vi "RetrievemeasurementByID.vi"(8 "error in (no error)":errorcluster, 10 "DatabaseConnectionInfo":T1, 11 "ID":string) -> (0 "error out":errorcluster, 1 "Variant data":variant[][](array[variant]), 2 "Double data":dbl[][](array[numeric]), 3 "String data":string[][](array[string]))   [LabVIEW 2017]
uses:
  <vilib>/addons/database/Connection.llb/DB Tools Open Connec (Path).vi
  <vilib>/addons/database/Connection.llb/Conn Execute.vi
  <vilib>/addons/database/Recordset.llb/Rec Fetch Recordset Data (R).vi
  <vilib>/addons/database/Recordset.llb/Rec Destroy - Connection.vi
  <vilib>/addons/database/_DB Variant To Data/Database Variant To Data.xnode
  <vilib>/addons/database/NI_Database_API.lvlib
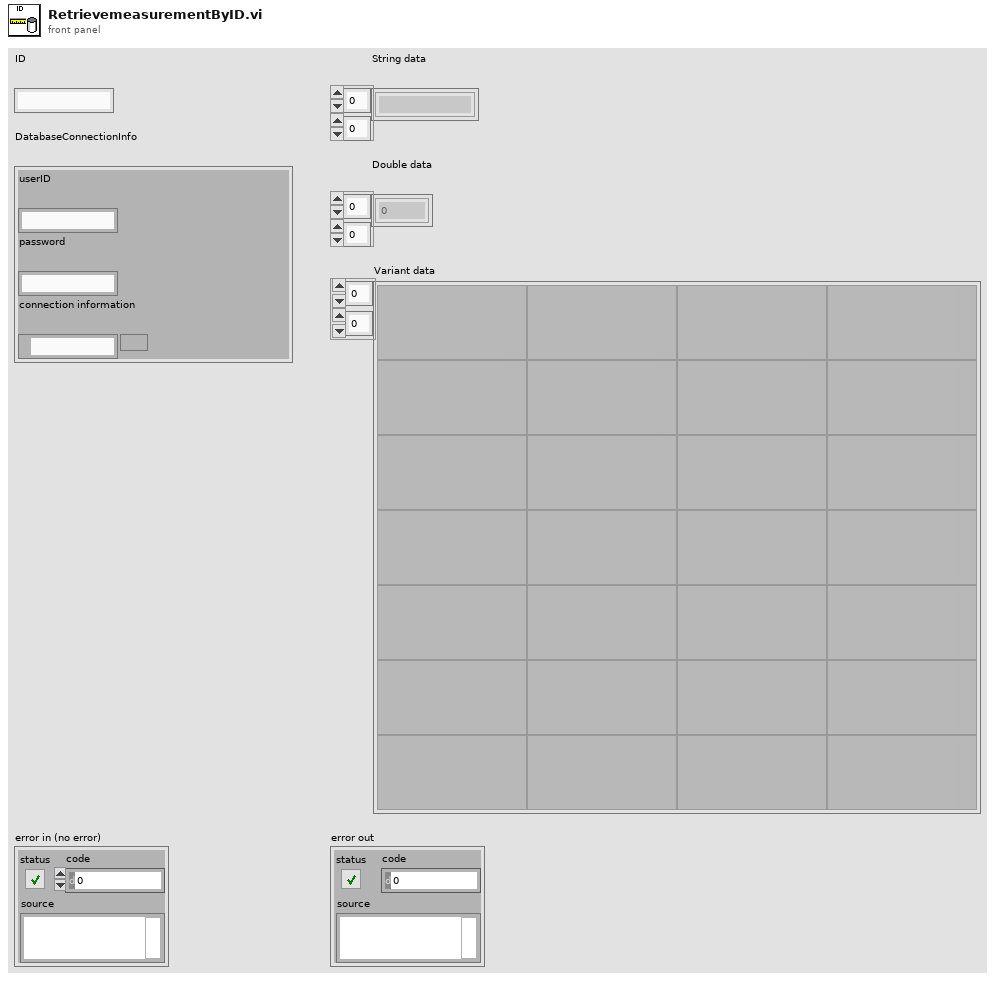
[diagram p1: front panel]
types:
  T1 = cluster{"userID":string, "password":string, "connection information":path}
  T2 = typedef "NI_Database_API.lvlib/Conn ObjectReference.ctl" = refnum<k1>
  T3 = typedef "NI_Database_API.lvlib/Rec ObjectReference.ctl" = refnum<k1>
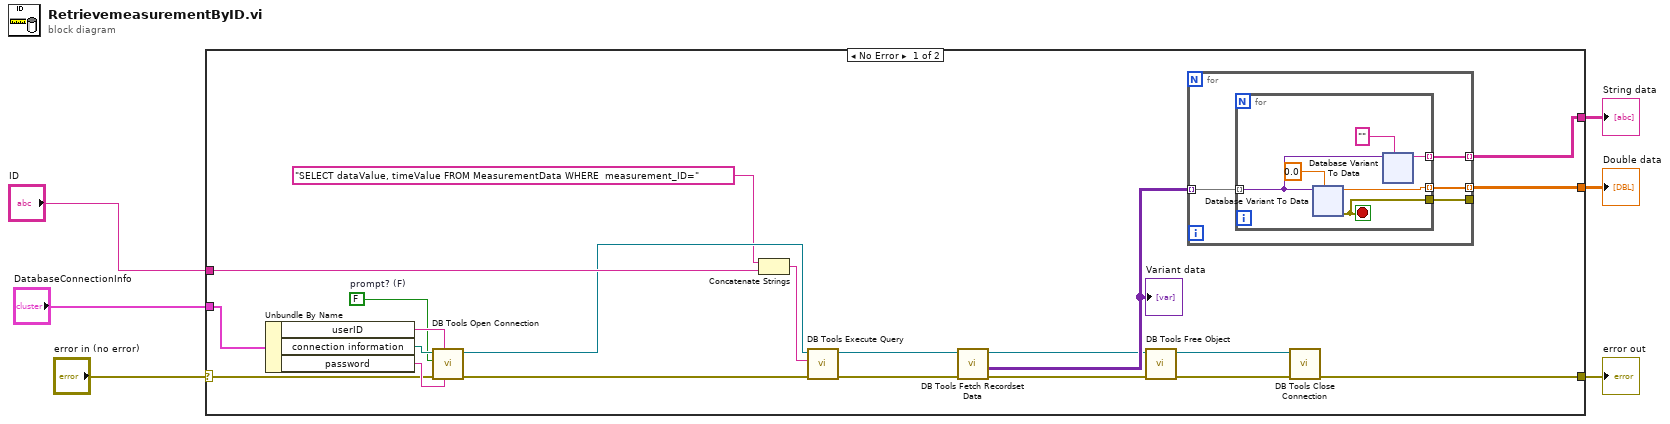
[diagram p0: block diagram]
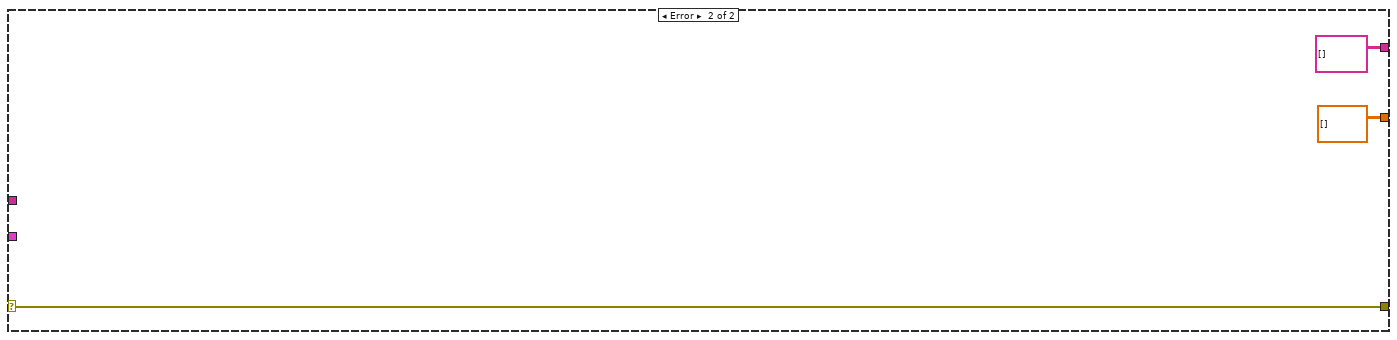
[diagram p2: hidden frame]
diagram:
  n1 = case shown="No Error" "error in (no error)" {
    selector: "error in (no error)" -> [w7 w104]
    tunnel: [w27 dbl[][] []] -> w6
    tunnel: [w26 string[][] []] -> w5
    tunnel: "ID" -> [w23 _]
    tunnel: "DatabaseConnectionInfo" -> [w22 _]
    tunnel: [w17 w104] -> w2
    frame No Error {
      w9 = FALSE  # prompt? (F)
      n2 = Unbundle By Name(w22) -> ("userID"=w10:string, "connection information"=w12:path, "password"=w11:string)
      n3 = call-poly <vilib>:"DB Tools Open Connection.vi"("password"=w11, "userID"=w10, "error in (no error)"=w7, "prompt? (F)"=w9, "connection information"=w12) -> ("error out"=w14:errorcluster, "connection reference"=w13:T2)  [unwired: 3 in]
      n4 = Concatenate Strings("SELECT dataValue, timeValue FROM MeasurementData WHERE  measurement_ID=", w23) -> (w24:string)
      n5 = call-poly <vilib>:"DB Tools Execute Query.vi"("error in (no error)"=w14, "SQL query"=w24, "connection reference"=w13) -> ("error out"=w21:errorcluster, "recordset reference"=w18:T3)  [unwired: 5 in]
      n6 = call-poly <vilib>:"DB Tools Fetch Recordset Data.vi"("error in (no error)"=w21, "recordset reference"=w18) -> ("error out"=w20:errorcluster, "recordset data"=w25:variant[][], "recordset reference out"=w19:T3)  [unwired: 3 in]
      "Variant data" <- w25
      n7 = call-poly <vilib>:"DB Tools Free Object.vi"("error in (no error)"=w20, "recordset reference"=w19) -> ("error out"=w16:errorcluster, "connection reference"=w15:T2)  [unwired: 8 in]
      n8 = for {
        tunnel: w25 -> [w31] mode=indexing
        tunnel: [w30] -> _
        tunnel: [w29] -> w27 mode=indexing
        tunnel: [w28] -> w26 mode=indexing
        n9 = for {
          tunnel: w31 -> [w34] mode=indexing
          tunnel: [w37] -> w30
          tunnel: [w36] -> w29 mode=indexing
          tunnel: [w32] -> w28 mode=indexing
          stop <- w37 stop-if-true
          n10 = xnode "Database Variant To Data"("database variant"=w34, "type"=0.0) -> ("data"=w36:dbl, "error out"=w37:errorcluster)  [unwired: 1 in]
          n11 = xnode "Database Variant To Data"("database variant"=w34, "type"="") -> ("data"=w32:string)  [unwired: 1 in, 1 out]
        }
      }
      n12 = call <vilib>:"DB Tools Close Connection.vi"("error in (no error)"=w16, "connection reference"=w15) -> ("error out"=w17:errorcluster)  [unwired: 5 in]
    }
    frame Error {
    }
  }
  "Double data" <- w6
  "String data" <- w5
  "error out" <- w2
